vi "free usb.vi"   [LabVIEW 2018, in "Dll1_x64_191014_0.lvlib"]
doc: "__declspec(dllexport) void free_usb();"
uses:
  Dll1_x64_191014_0.lvlib
  Dll1.dll
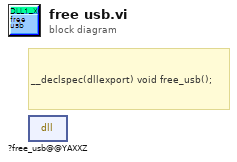
[diagram p0: block diagram]
diagram:
  # "__declspec(dllexport) void free_usb();"
  n1 = dll-call lib="PTH2zabs CUsersLenovoDesktopDHCC실험2#lux image capture_0.9.1.1_Temporaryuser.libDll1_x64_191014_0Dll1.*" fn="?free_usb@@YAXXZ"() -> ()  [unwired: 4 in, 2 out]
